vi "Handle Modules Change.vi"(7 "Modules Page Controls":T3, 8 "error in (no error)":errorcluster, 9 "NewVal":T2[](array[typedef]), 10 "OldVal":T2[](array[typedef]), 11 "Routing and Faulting Ref in":T1 format="%.0x") -> (0 "error out":errorcluster, 3 "Routing and Faulting Ref out":T1 format="%.0x")   [LabVIEW 2017, in "Routing and Faulting System Explorer.lvlib"]
uses:
  Routing and Faulting System Explorer.lvlib
  Modules Page Controls.ctl
  Module Row.ctl
  <vilib>/NI Veristand/Custom Device API/Custom Device Item Ref.ctl
  NationalInstruments.VeriStand.SystemStorage
  Shared/Routing and Faulting Hardware API/Routing and Faulting Hardware API.lvlib
  <vilib>/NI Veristand/Custom Device API/Custom Device API.lvlib
  Scripting/Routing and Faulting Scripting.lvlib
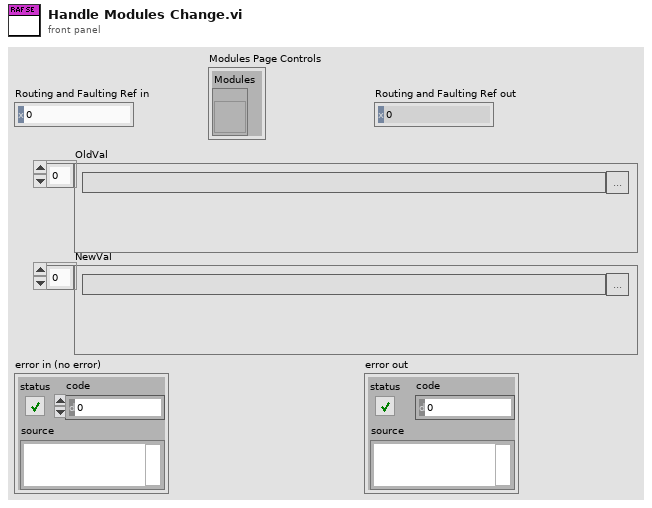
[diagram p1: front panel]
types:
  T1 = typedef "Custom Device API.lvlib/Custom Device Item Ref.ctl" = u64
  T2 = typedef "Routing and Faulting System Explorer.lvlib/Module Row.ctl" = cluster{"Module path":string, "Edit":bool, "Description":string}
  T3 = typedef "Modules Page Controls.ctl" = cluster{"Modules":refnum<vi>}
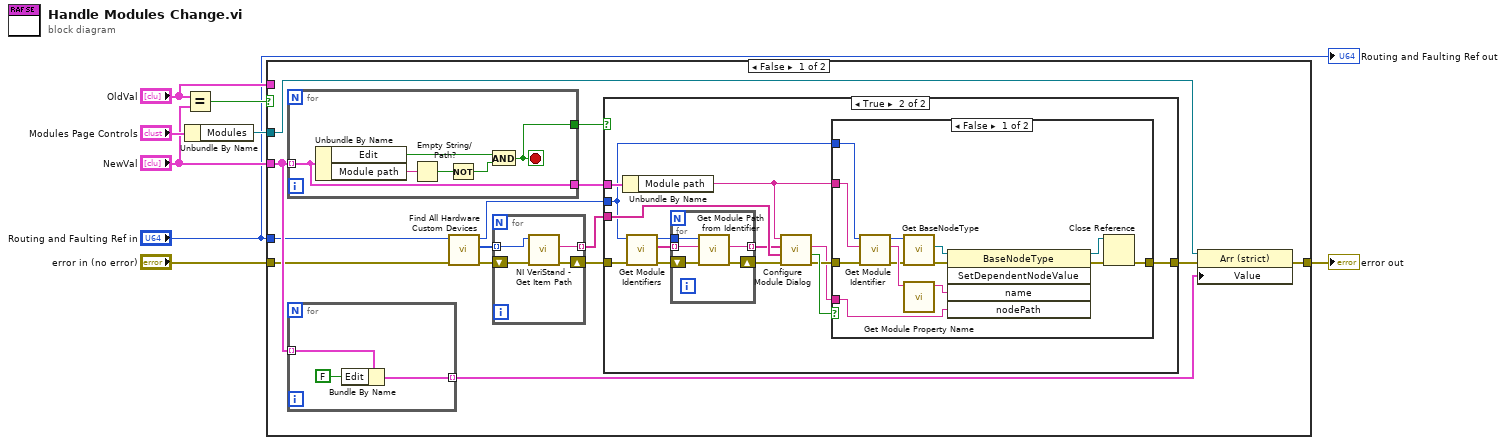
[diagram p0: block diagram]
diagram:
  n1 = Equal?(x="OldVal", y="NewVal") -> (x = y?=w4:bool)
  n2 = Unbundle By Name("Modules Page Controls") -> ("Modules"=w8:refnum<vi>)
  n3 = case shown="False" w4 {
    tunnel: "OldVal" -> [_ _]
    tunnel: "NewVal" -> [w19 _]
    tunnel: w8 -> [w20 _]
    tunnel: "error in (no error)" -> [w16 w70]
    tunnel: [w17 w70] -> w2
    tunnel: "Routing and Faulting Ref in" -> [w15 _]
    frame False {
      n4 = for {
        tunnel: w19 -> [w69] mode=indexing
        tunnel: [w69] -> w21
        tunnel: [w64] -> w22
        stop <- w64 stop-if-true
        n5 = Unbundle By Name(w69) -> ("Edit"=w68:bool, "Module path"=w67:string)
        n6 = Empty String/Path?(string/path=w67) -> (empty?=w66:bool)
        n7 = Not(x=w66) -> (.not. x?=w65:bool)
        n8 = And(x=w68, y=w65) -> (x .and. y?=w64:bool)
      }
      n9 = for {
        tunnel: w19 -> [w29] mode=indexing
        tunnel: [w27] -> w18 mode=indexing
        n10 = Bundle By Name(cluster=w29, "Edit"=FALSE) -> (w27:T2)
      }
      n11 = call "Find All Hardware Custom Devices.vi"("error in (no error)"=w16, "Routing and Faulting Ref in"=w15) -> ("error out"=w14:errorcluster, "Hardware Refs"=w12:T1[], "Routing and Faulting Ref out"=w9:T1)  [unwired: 7 in]
      n12 = for {
        tunnel: w12 -> [w26] mode=indexing
        shift-right: [w24] -> w11
        shift-left: w14 -> [w25]
        tunnel: [w23] -> w13 mode=indexing
        n13 = call <vilib>:"NI VeriStand - Get Item Path.vi"("error in (no error)"=w25, "Item Ref in"=w26) -> ("error out"=w24:errorcluster, "Path"=w23:string)  [unwired: 6 in, 2 out]
      }
      n14 = case shown="True" w22 {
        tunnel: w21 -> [_ w44]
        tunnel: w13 -> [_ w38]
        tunnel: w11 -> [w30 w37]
        tunnel: [w30 w41] -> w10
        tunnel: w9 -> [_ w36]
        frame False {
        }
        frame True {
          n15 = Unbundle By Name(w44) -> ("Module path"=w39:string)
          n16 = call "Get Module Identifiers.vi"("error in (no error)"=w37, "Routing and Faulting Ref in"=w36) -> ("error out"=w34:errorcluster, "Module Identifiers"=w35:string[], "Routing and Faulting Ref out"=w33:T1)  [unwired: 7 in]
          n17 = for {
            tunnel: w35 -> [w49] mode=indexing
            tunnel: w33 -> [w47]
            shift-right: [w46] -> w32
            shift-left: w34 -> [w48]
            tunnel: [w45] -> w31 mode=indexing
            n18 = call "Get Module Path from Identifier.vi"("error in (no error)"=w48, "Module identifier"=w49, "Routing and Faulting Ref in"=w47) -> ("error out"=w46:errorcluster, "Module path"=w45:string)  [unwired: 6 in, 1 out]
          }
          n19 = call "Configure Module Dialog.vi"("error in (no error)"=w32, "Possible Modules"=w38, "Existing Modules"=w31, "Source"=w39) -> ("error out"=w42:errorcluster, "Canceled?"=w43:bool, "New Module Path"=w40:string)  [unwired: 5 in]
          n20 = case shown="False" w43 {
            tunnel: w42 -> [w62 w63]
            tunnel: w36 -> [w61 _]
            tunnel: w39 -> [w60 _]
            tunnel: [w56 w63] -> w41
            tunnel: w40 -> [w54 _]
            frame False {
              n21 = call "Get Module Identifier.vi"("error in (no error)"=w62, "Module path"=w60, "Routing and Faulting Ref in"=w61) -> ("error out"=w51:errorcluster, "Module identifier"=w59:string, "Routing and Faulting Ref out"=w53:T1)  [unwired: 5 in, 1 out]
              n22 = call "Get BaseNodeType.vi"("error in (no error)"=w51, "Item Ref in"=w53) -> ("error out"=w52:errorcluster, "BaseNodeType"=w50:refnum<k24>)  [unwired: 7 in, 1 out]
              n23 = call "Get Module Property Name.vi"("Module ID"=w59) -> ("Module Property Name"=w55:string)  [unwired: 10 in]
              n24 = invoke class="BaseNodeType" method="SetDependentNodeValue"(reference=w50, error in=w52, "name"=w55, "nodePath"=w54) -> (reference out=w57:refnum<k24>, error out=w58:errorcluster)  [unwired: 1 in, 3 out]
              n25 = Close Reference(reference=w57, error in (no error)=w58) -> (error out=w56:errorcluster)
            }
            frame True {
            }
          }
        }
      }
      n26 = property class="Arr (strict)"(reference=w20, error in=w10, "Value"=w18) -> (error out=w17:errorcluster)  [unwired: 1 out]
    }
    frame True {
    }
  }
  "error out" <- w2
  "Routing and Faulting Ref out" <- "Routing and Faulting Ref in"
